vi "ParameterCfgLoad.vi"(2 "Section":string, 3 "configuration file path":path) -> (0 "section names list":string[](array[string]), 1 "Array - String":string[][](array[string]))   [LabVIEW 2019]
uses:
  <vilib>/Utility/config.llb/Read Key (String).vi
  <vilib>/Utility/config.llb/NI_LVConfig.lvlib
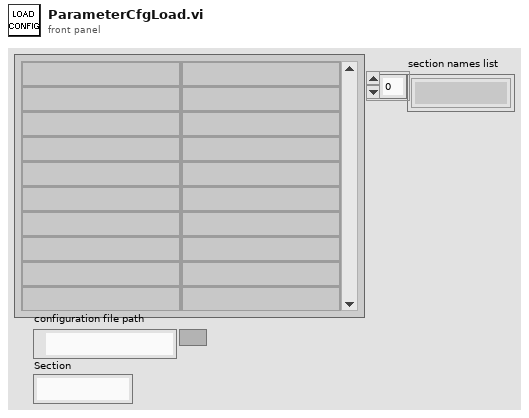
[diagram p1: front panel]
types:
  T1 = typedef "NI_LVConfig.lvlib/Config Data RefNum.ctl" = refnum<k1>
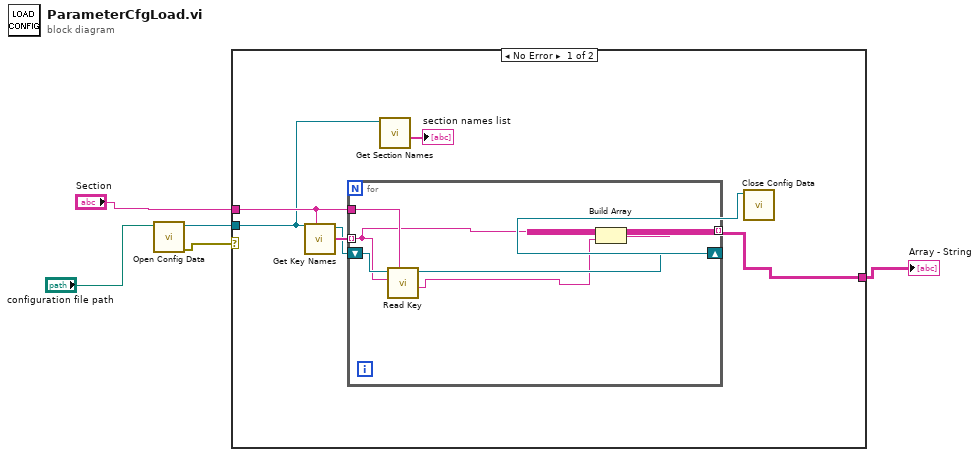
[diagram p0: block diagram]
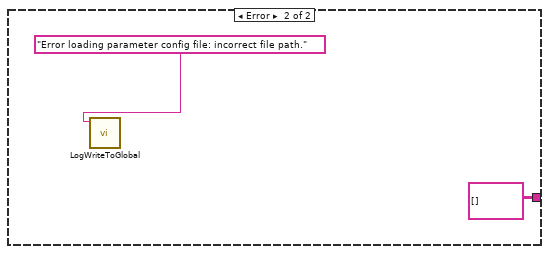
[diagram p2: hidden frame]
diagram:
  n1 = call <vilib>:"Open Config Data.vi"("configuration file path"="configuration file path") -> ("error out"=w1:errorcluster, "refnum"=w3:T1)  [unwired: 8 in, 1 out]
  n2 = case shown="No Error" w1 {
    tunnel: "Section" -> [w9 _]
    tunnel: w3 -> [w8 _]
    tunnel: [w6 string[][] []] -> w2
    frame No Error {
      n3 = call <vilib>:"Get Key Names.vi"("section"=w9, "refnum"=w8) -> ("key names"=w12:string[], "refnum out"=w11:T1)  [unwired: 6 in, 2 out]
      n4 = for {
        tunnel: w12 -> [w16] mode=indexing
        tunnel: w9 -> [w17]
        tunnel: [w15] -> w6 mode=indexing
        shift-right: [w14] -> w10
        shift-left: w11 -> [w18]
        n5 = call-poly <vilib>:"Read Key.vi"("section"=w17, "key"=w16, "refnum"=w18) -> ("value"=w13:string, "refnum out"=w14:T1)  [unwired: 5 in, 2 out]
        n6 = Build Array(w16, w13) -> (w15:string[])
      }
      n7 = call <vilib>:"Get Section Names.vi"("refnum"=w8) -> ("section names"=→"section names list":string[])  [unwired: 8 in, 2 out]
      n8 = call <vilib>:"Close Config Data.vi"("refnum"=w10) -> ()  [unwired: 9 in, 2 out]
    }
    frame Error {
      n9 = call "LogWriteToGlobal.vi"("in string"="Error loading parameter config file: incorrect file path.") -> ()  [unwired: 11 in]
    }
  }
  "Array - String" <- w2
